vi "Write elementFactory.vi"(10 "IElementFactory.lvclass":refnum<class "IElementFactory.lvclass">, 11 "Topic in":refnum<class "Topic.lvclass">) -> (3 "Topic out":refnum<class "Topic.lvclass">)   [LabVIEW 2016, in "Topic.lvclass"]
uses:
  Topic.lvclass
  ElementFactory/IElementFactory/IElementFactory.lvclass
  Topic.lvclass/Topic.ctl
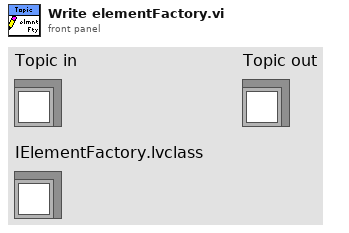
[diagram p1: front panel]
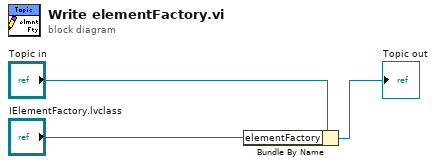
[diagram p0: block diagram]
diagram:
  n1 = Bundle By Name(cluster="Topic in", "elementFactory"="IElementFactory.lvclass") -> (→"Topic out":refnum<class "Topic.lvclass">)
